vi "Cavities_Pulse_FPGA_v00.vi"() -> ()   [LabVIEW 2010]
doc: "Four cavities are controlled here:\n1) OPO A\n2) OPO B\n3) mode Cleaner\n4) Doubler\nThe output can either be Scanned, Locked, or Held."
uses:
  Strict Type Defs/Scope.ctl
  Strict Type Defs/Pulse Control.ctl
  Strict Type Defs/Cavity Errors.ctl
  Strict Type Defs/Cavity Monitors.ctl
  Strict Type Defs/Zero Crossing.ctl
  Strict Type Defs/Control.ctl
  Strict Type Defs/PII individual.ctl
  Strict Type Defs/Safety First.ctl
  Strict Type Defs/Error Scale.ctl
  Strict Type Defs/Lock Thresh.ctl
  <vilib>/eio/EIONode/EIONode.xnode
  <vilib>/rvi/eio/nirviEIOImplementation/nirviEIOImplementation.xnode
  <vilib>/rvi/eio/common/nirviEmuClasses.ctl
  <vilib>/rvi/DataTransferAndStorage/Container/XNode/niFpgaContainer.xnode
  <vilib>/rvi/DataTransferAndStorage/Container/Common/niFpgaContainerMethod.ctl
  <vilib>/rvi/DataTransferAndStorage/Container/Common/niFpgaTransferTypeControl.ctl
  <vilib>/rvi/eio/common/nirviEmuTemplateMethod_noerrors.vi
  <vilib>/rvi/interface/RandomDataEmulation/nirviRandomDataFPGAFIFO.vi
  <vilib>/rvi/interface/RandomDataEmulation/niFpgaRandomDataHandleErrors.vi
panel:
  in  "quit Control Loop":bool
  in  "Control":T1={"PII In 1"={"Lock"=FALSE, "Hold"=FALSE, "P Gain"=0, "P BS"=-5, "I Gain"=0, "I BS"=-10, "I2 G"=0, "I2 BS"=-26, "Scan Amp"=0, "Scan Off"=0, "Scan FS"=0, "SFS BS"=0, "I Max value"=10000, "I2 Max value"=10000, "Scope.Offset"=0, "Trigger Direction"=enum."either", "Scan-PII thresh"=0}, "PII In 2"={"Lock"=FALSE, "Hold"=FALSE, "P Gain"=0, "P BS"=-10, "I Gain"=0, "I BS"=-10, "I2 G"=0, "I2 BS"=-26, "Scan Amp"=0, "Scan Off"=0, "Scan FS"=0, "SFS BS"=0, "I Max value"=10000, "I2 Max value"=10000, "Scope.Offset"=0, "Trigger Direction"=enum."either", "Scan-PII thresh"=0}, "PII In 3"={"Lock"=FALSE, "Hold"=FALSE, "P Gain"=0, "P BS"=-10, "I Gain"=0, "I BS"=-10, "I2 G"=0, "I2 BS"=-26, "Scan Amp"=0, "Scan Off"=0, "Scan FS"=0, "SFS BS"=0, "I Max value"=10000, "I2 Max value"=10000, "Scope.Offset"=0, "Trigger Direction"=enum."either", "Scan-PII thresh"=0}, "PII In 4"={"Lock"=FALSE, "Hold"=FALSE, "P Gain"=0, "P BS"=-10, "I Gain"=0, "I BS"=-10, "I2 G"=0, "I2 BS"=-26, "Scan Amp"=0, "Scan Off"=0, "Scan FS"=0, "SFS BS"=0, "I Max value"=10000, "I2 Max value"=10000, "Scope.Offset"=0, "Trigger Direction"=enum."either", "Scan-PII thresh"=0}, "Safety First"={"lim reset"=FALSE, "no limit"=FALSE, "pos slew rate * dt"=10, "neg slew rate * dt"=-10, "Hold All"=FALSE, "Count(Ticks)"=0}, "Error scale"={"Pre-Offset"={"Pre-Offset 1"=2, "Pre-Offset 2"=0, "Pre-Offset 3"=0, "Pre-Offset 4"=0, "Pre-Offset 5"=2, "Pre-Offset 6"=0, "Pre-Offset 7"=0, "Pre-Offset 8"=0}, "Post-Offset "={"Offset 1"=0, "Offset 2"=300, "Offset 3"=0, "Offset 4"=0, "Offset 5"=0, "Offset 6"=0, "Offset 7"=0, "Offset 8"=0}, "Gains"={"Gain 1"=0, "Gain 2"=300, "Gain 3"=0, "Gain 4"=0, "Gain 5"=0, "Gain 6"=0, "Gain 7"=0, "Gain 8"=0}, "Polarity DC"={"False 1"=FALSE, "False 2"=FALSE, "False 3"=FALSE, "False 4"=FALSE, "DC x -1"=FALSE, "DC x -1 2"=FALSE, "DC x -1 3"=FALSE, "DC x -1 4"=FALSE}}, "Lock Thresh"={"OPO A"=2, "OPO B"=0, "MCC"=40, "Doubler"=0}, "Re-Scan Thresh"={"OPO A"=0, "OPO B"=0, "MCC"=0, "Doubler"=0}}
  in  "\"I too high?\"":T6
  in  "\"Outputs\"":T7
  out "Outputs":T8={"OPO A out"=-270, "OPO B out"=-1710, "MCC out"=880, "Doubler out"=570}
  in  "\"Trigger\"":T9
  out "Trigger":T9
  out "Cavity Monitors":T10
  out "Cavity Errors":T11={"OPO A"=0, "OPO B"=1800, "MCC"=0, "Doubler"=0}
  out "Control Loop count":i32=11285327
  out "Lock Threshold":T12
  in  "Cavities Delay(uSec)":u32 caption="Count(uSec)"
  in  "Lock Monitor":T7
  out "Unlocked?(T=yes)":T6
  in  "RMS Stop":bool
  out "RMS Count":i32
  in  "Measurement OFF (uSec)":u32 caption="Measurement OFF(uSec)"
  in  "offset time":u32
  out "Measurement Tick Count(uSec)":u32
  out "PXI Trig 2":bool
  in  "Measurement OFF":bool
  out "Pulse large loop count":i32
  in  "Pulse Loop On":bool
  in  "stop pulse loop":bool
  out "Pulse Loop count":i32
  out "Tick Count(uSec)":u32
  out "BS Hold Pulse":bool
  out "Probe OFF Pulse":bool
  out "HD Pulse":bool
  out "Measurment Pulse":bool
  in  "Pulse Control":T13
  in  "Scope":T14={"Trigger Direction"=enum."plus-minus", "Delay"=0, "Aquisition Rate (Ticks)"=40, "Offset"=0, "Channel"=0, "Channel Selector"={"Channel 1"=0, "Channel 2"=4, "Channel 3"=8, "Channel 4"=8}} {"Channel Selector"."Channel 4" items=["Error Signal 1", "Error Signal 2", "Scan Trigger 1", "Scan Trigger 2", "DC Signal 1", "DC Signal 2", "PI Out 1", "PI Out 2"]; "Channel Selector"."Channel 3" items=["Error Signal 1", "Error Signal 2", "Scan Trigger 1", "Scan Trigger 2", "DC Signal 1", "DC Signal 2", "PI Out 1", "PI Out 2"]; "Channel Selector"."Channel 2" items=["Error Signal 1", "Error Signal 2", "Scan Trigger 1", "Scan Trigger 2", "DC Signal 1", "DC Signal 2", "PI Out 1", "PI Out 2"]; "Channel Selector"."Channel 1" items=["Error Signal 1", "Error Signal 2", "Scan Trigger 1", "Scan Trigger 2", "DC Signal 1", "DC Signal 2", "PI Out 1", "PI Out 2"]}
  out "Scope Full?":bool
  out "Scope loop count":i32=119818
  # "All time values are in micro-seconds"
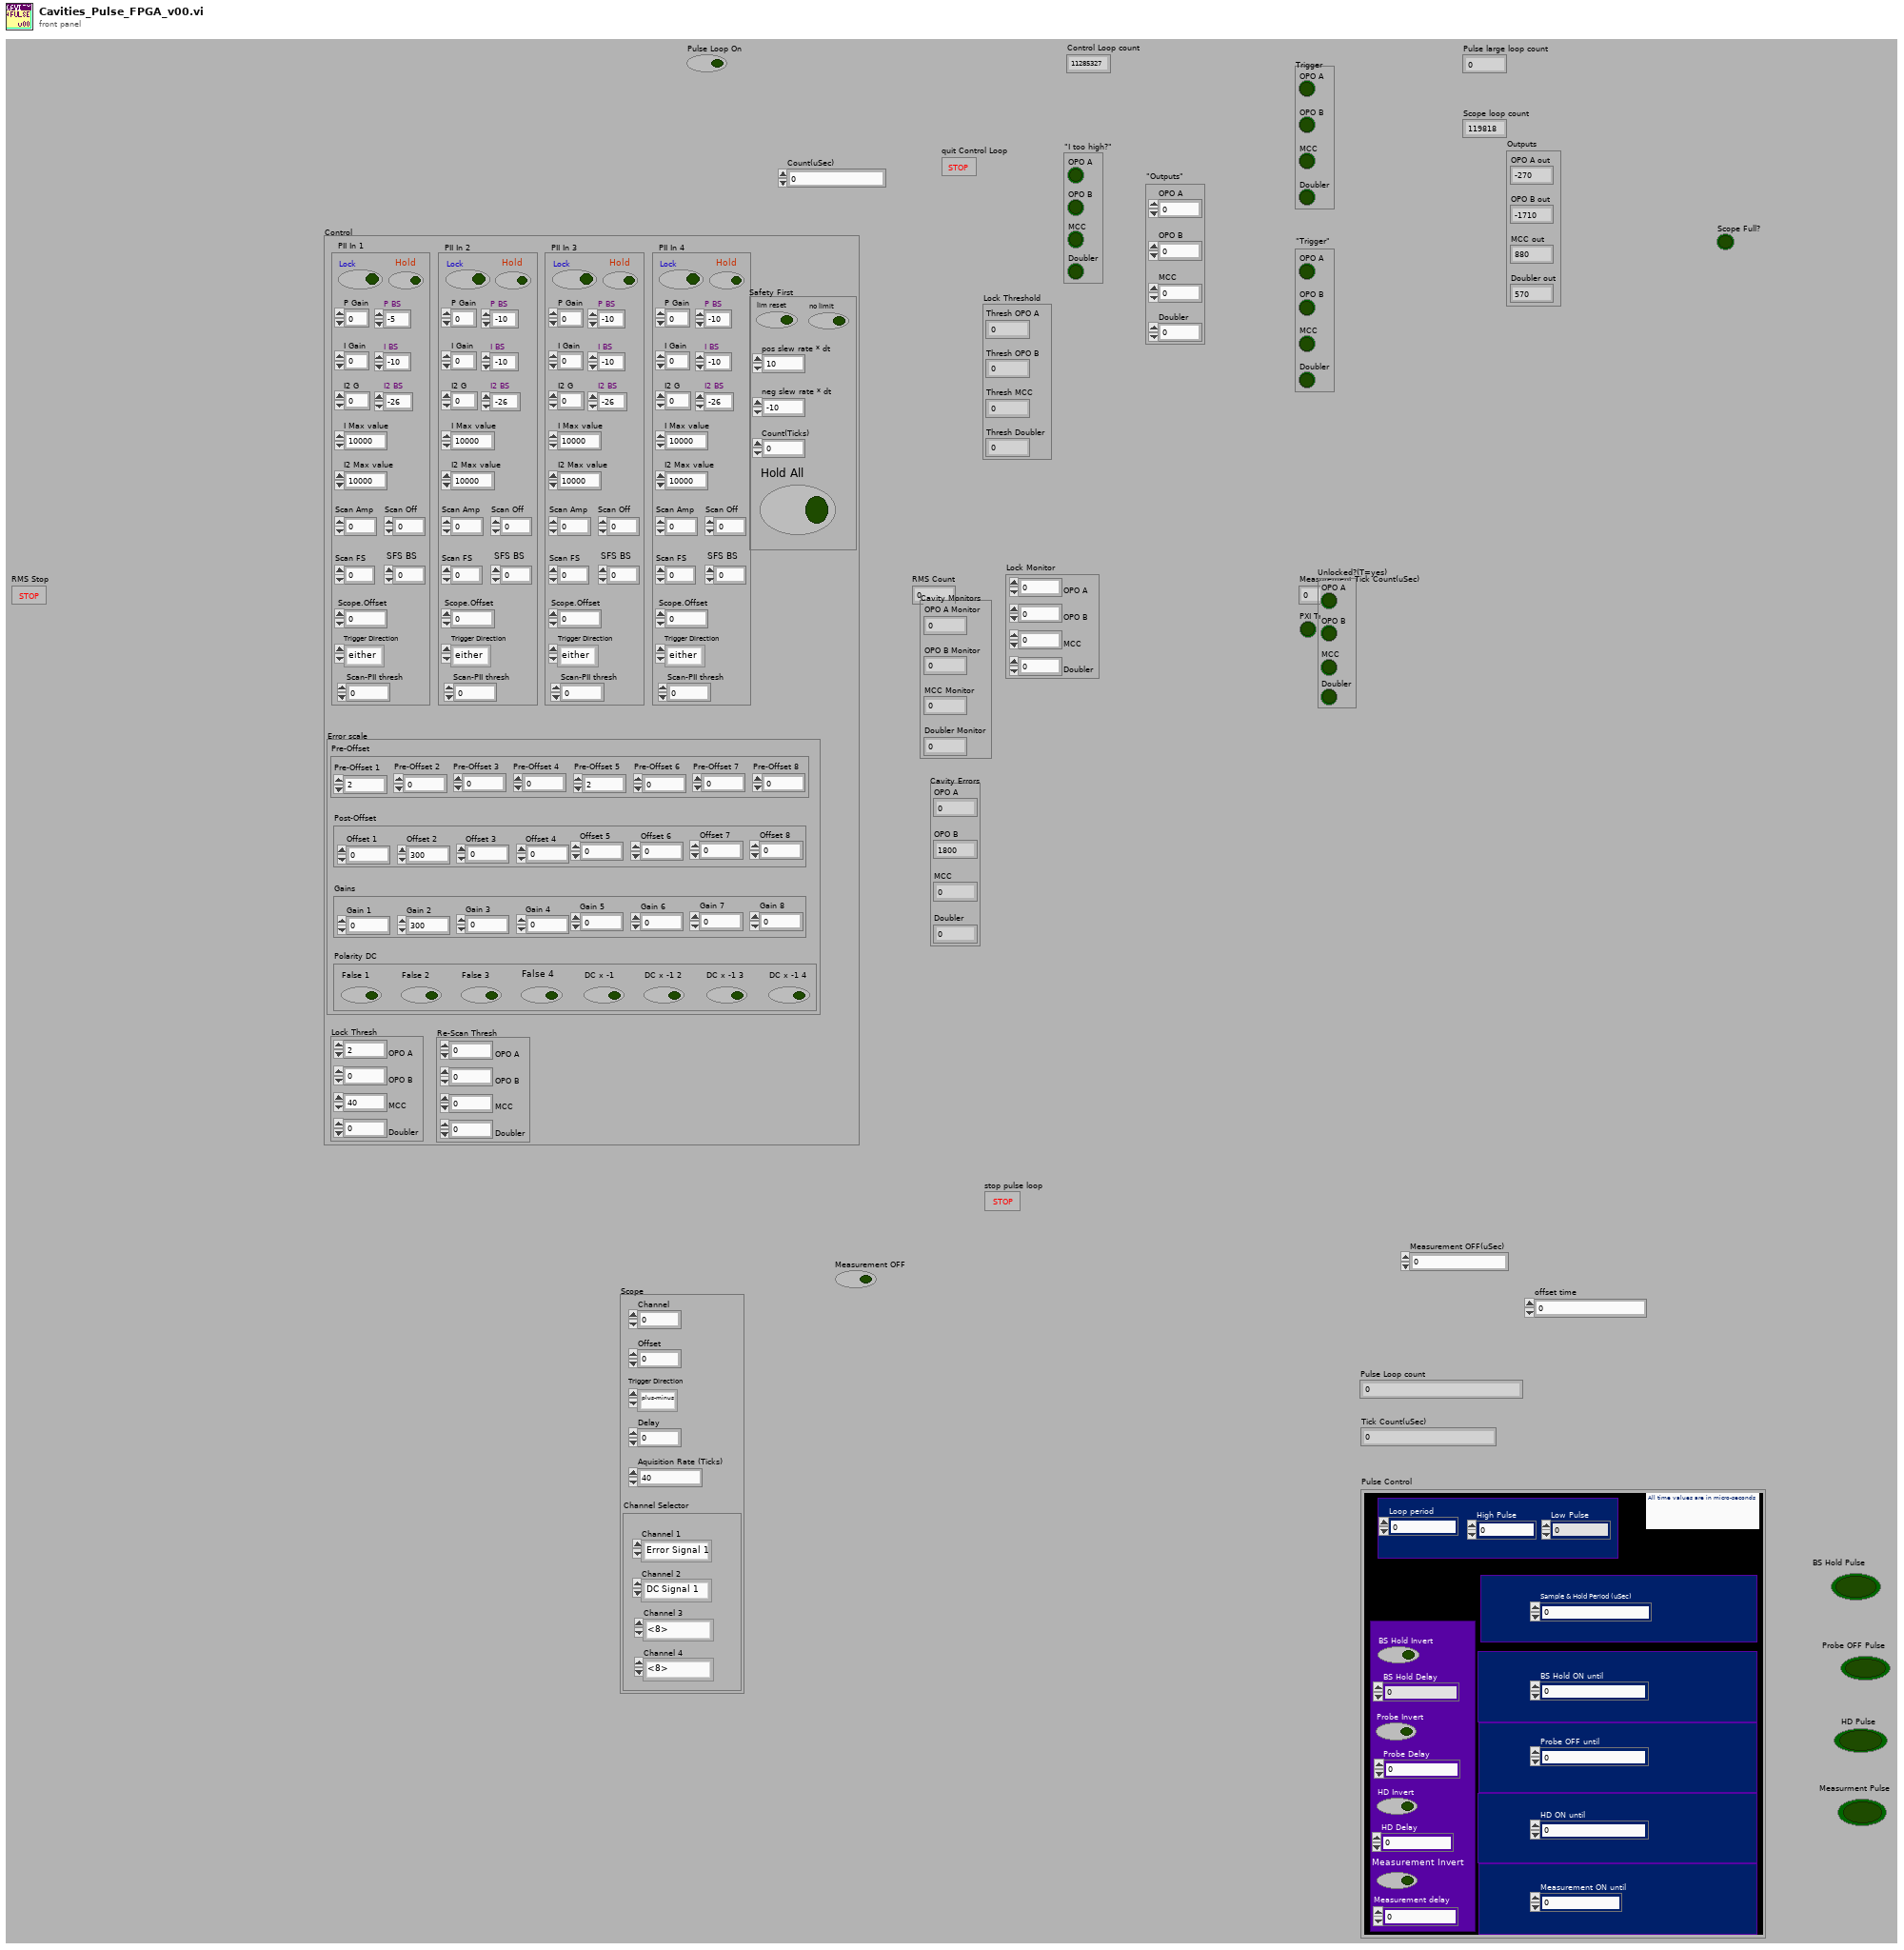
[diagram p1: front panel]
types:
  T1 = typedef "Control.ctl" = cluster{"PII In 1":T2, "PII In 2":T2, "PII In 3":T2, "PII In 4":T2, "Safety First":T3, "Error scale":T4, "Lock Thresh":T5, "Re-Scan Thresh":T5}
  T2 = typedef "PII individual.ctl" = cluster{"Lock":bool, "Hold":bool, "P Gain":i32, "P BS":i16, "I Gain":i32, "I BS":i16, "I2 G":i32, "I2 BS":i16, "Scan Amp":i16, "Scan Off":i16, "Scan FS":u16, "SFS BS":i16, "I Max value":i32, "I2 Max value":i32, "Scope.Offset":i16, "Trigger Direction":enum8{"either", "minus-plus", "plus-minus"}, "Scan-PII thresh":i16}
  T3 = typedef "Safety First.ctl" = cluster{"lim reset":bool, "no limit":bool, "pos slew rate * dt":i16, "neg slew rate * dt":i16, "Hold All":bool, "Count(Ticks)":u32}
  T4 = typedef "Error Scale.ctl" = cluster{"Pre-Offset":cluster{"Pre-Offset 1":i16, "Pre-Offset 2":i16, "Pre-Offset 3":i16, "Pre-Offset 4":i16, "Pre-Offset 5":i16, "Pre-Offset 6":i16, "Pre-Offset 7":i16, "Pre-Offset 8":i16}, "Post-Offset ":cluster{"Offset 1":i16, "Offset 2":i16, "Offset 3":i16, "Offset 4":i16, "Offset 5":i16, "Offset 6":i16, "Offset 7":i16, "Offset 8":i16}, "Gains":cluster{"Gain 1":i16, "Gain 2":i16, "Gain 3":i16, "Gain 4":i16, "Gain 5":i16, "Gain 6":i16, "Gain 7":i16, "Gain 8":i16}, "Polarity DC":cluster{"False 1":bool, "False 2":bool, "False 3":bool, "False 4":bool, "DC x -1":bool, "DC x -1 2":bool, "DC x -1 3":bool, "DC x -1 4":bool}}
  T5 = typedef "Lock Thresh.ctl" = cluster{"OPO A":i16, "OPO B":i16, "MCC":i16, "Doubler":i16}
  T6 = cluster{"OPO A":bool, "OPO B":bool, "MCC":bool, "Doubler":bool}
  T7 = cluster{"OPO A":i16, "OPO B":i16, "MCC":i16, "Doubler":i16}
  T8 = cluster{"OPO A out":i16, "OPO B out":i16, "MCC out":i16, "Doubler out":i16}
  T9 = typedef "Zero Crossing.ctl" = cluster{"OPO A":bool, "OPO B":bool, "MCC":bool, "Doubler":bool}
  T10 = typedef "Cavity Monitors.ctl" = cluster{"OPO A Monitor":i16, "OPO B Monitor":i16, "MCC Monitor":i16, "Doubler Monitor":i16}
  T11 = typedef "Cavity Errors.ctl" = cluster{"OPO A":i16, "OPO B":i16, "MCC":i16, "Doubler":i16}
  T12 = cluster{"Thresh OPO A ":i16, "Thresh OPO B":i16, "Thresh MCC":i16, "Thresh Doubler":i16}
  T13 = typedef "Pulse Control.ctl" = cluster{"BS Hold Invert":bool, "Probe Invert":bool, "HD Invert":bool, "Measurement Invert":bool, "BS Hold Delay":u32, "Probe Delay":u32, "HD Delay":u32, "Measurement delay":u32, "High Pulse":i16, "Low Pulse":i16, "Sample & Hold Period (uSec)":u32, "BS Hold ON until":u32, "Probe OFF until":u32, "HD ON until":u32, "Measurement ON until":u32, "Loop period (us)":u16}
  T14 = typedef "Scope.ctl" = cluster{"Trigger Direction":enum8{"either", "minus-plus", "plus-minus"}, "Delay":u32, "Aquisition Rate (Ticks)":u32, "Offset":i16, "Channel":i32, "Channel Selector":cluster{"Channel 1":i32, "Channel 2":i32, "Channel 3":i32, "Channel 4":i32}}
  T15 = typedef "nirviEmuClasses.ctl" = enum16{"IO Read", "IO Write", "Method", "Property Read", "Property Write"}
  T16 = typedef "Signals.ctl" = cluster{"Cavity Errors":T11, "Cavity Monitors":T10, "Lock Thresh":T5, "Re-Scan Thresh":T5, "PII In 1":T2, "PII In 2":T2, "PII In 3":T2, "PII In 4":T2, "Safety First":T3}
  T17 = typedef "Control Cavity Cluster.ctl" = cluster{"Control A":T2, "Control B":T2, "Control MCC":T2, "Control Doubler":T2, "Lock Point?":T18, "Re-scan?":T19, "Cavity Errors":T11, "Max":T20, "Min":T21, "Lock Threshold":cluster{"Thresh OPO A ":i16, "Thresh OPO B":i16, "Thresh MCC":i16, "Thresh Doubler":i16}, "Re-Scan Threshold":cluster{"Thresh OPO A ":i16, "Thresh OPO B":i16, "Thresh MCC":i16, "Thresh Doubler":i16}, "State (-1)":cluster{"OPO A":enum16{"Safe", "Hold", "Scan", "Lock"}, "OPO B":enum16{"Safe", "Hold", "Scan", "Lock"}, "MCC":enum16{"Safe", "Hold", "Scan", "Lock"}, "Doubler":enum16{"Safe", "Hold", "Scan", "Lock"}}, "Lock pressed? (-1)":cluster{"OPO A":bool, "OPO B":bool, "MCC":bool, "Doubler":bool}, "Safety First":T3}
  T18 = typedef "Lock Point.ctl" = cluster{"OPO A":bool, "OPO B":bool, "MCC":bool, "Doubler":bool}
  T19 = typedef "Re-Scan.ctl" = cluster{"OPO A":bool, "OPO B":bool, "MCC":bool, "Doubler":bool}
  T20 = typedef "Max.ctl" = cluster{"Max OPO A":i16, "Max OPO B":i16, "Max MCC":i16, "Max Doubler":i16}
  T21 = typedef "Min.ctl" = cluster{"Min OPO A":i16, "Min OPO B":i16, "Min MCC":i16, "Min Doubler":i16}
  T22 = typedef "PII Scan State.ctl" = cluster{"Control A":T2, "Control B":T2, "Control MCC":T2, "Control Doubler":T2, "Cavity Errors":T11, "State":cluster{"OPO A":enum16{"Safe", "Hold", "Scan", "Lock"}, "OPO B":enum16{"Safe", "Hold", "Scan", "Lock"}, "MCC":enum16{"Safe", "Hold", "Scan", "Lock"}, "Doubler":enum16{"Safe", "Hold", "Scan", "Lock"}}}
  T23 = typedef "MaxMin.ctl" = cluster{"State":cluster{"OPO A":enum16{"Safe", "Hold", "Scan", "Lock"}, "OPO B":enum16{"Safe", "Hold", "Scan", "Lock"}, "MCC":enum16{"Safe", "Hold", "Scan", "Lock"}, "Doubler":enum16{"Safe", "Hold", "Scan", "Lock"}}, "Reset MaxMin?":cluster{"OPO A":bool, "OPO B":bool, "MCC":bool, "Doubler":bool}, "Max":T20, "Min":T21, "Lock pressed?":cluster{"OPO A":bool, "OPO B":bool, "MCC":bool, "Doubler":bool}, "Safety First":T3}
  T24 = typedef "niFpgaContainerMethod.ctl" = enum16{"<none>", "write", "read", "clear", "getNumberOfElementsToWrite", "getNumberOfElementsToRead", "enable", "disable", "flushAndDisable", "getStreamState", "readA", "readB", "dramWrite", "dramWriteWithByteEnables", "dramRequestData", "dramRetrieveData"}
  T25 = typedef "niFpgaTransferTypeControl.ctl" = enum16{"Target-Scoped", "Host to Target - DMA", "Target to Host - DMA", "Peer to Peer Reader", "Peer to Peer Writer", "Bidirectional"}
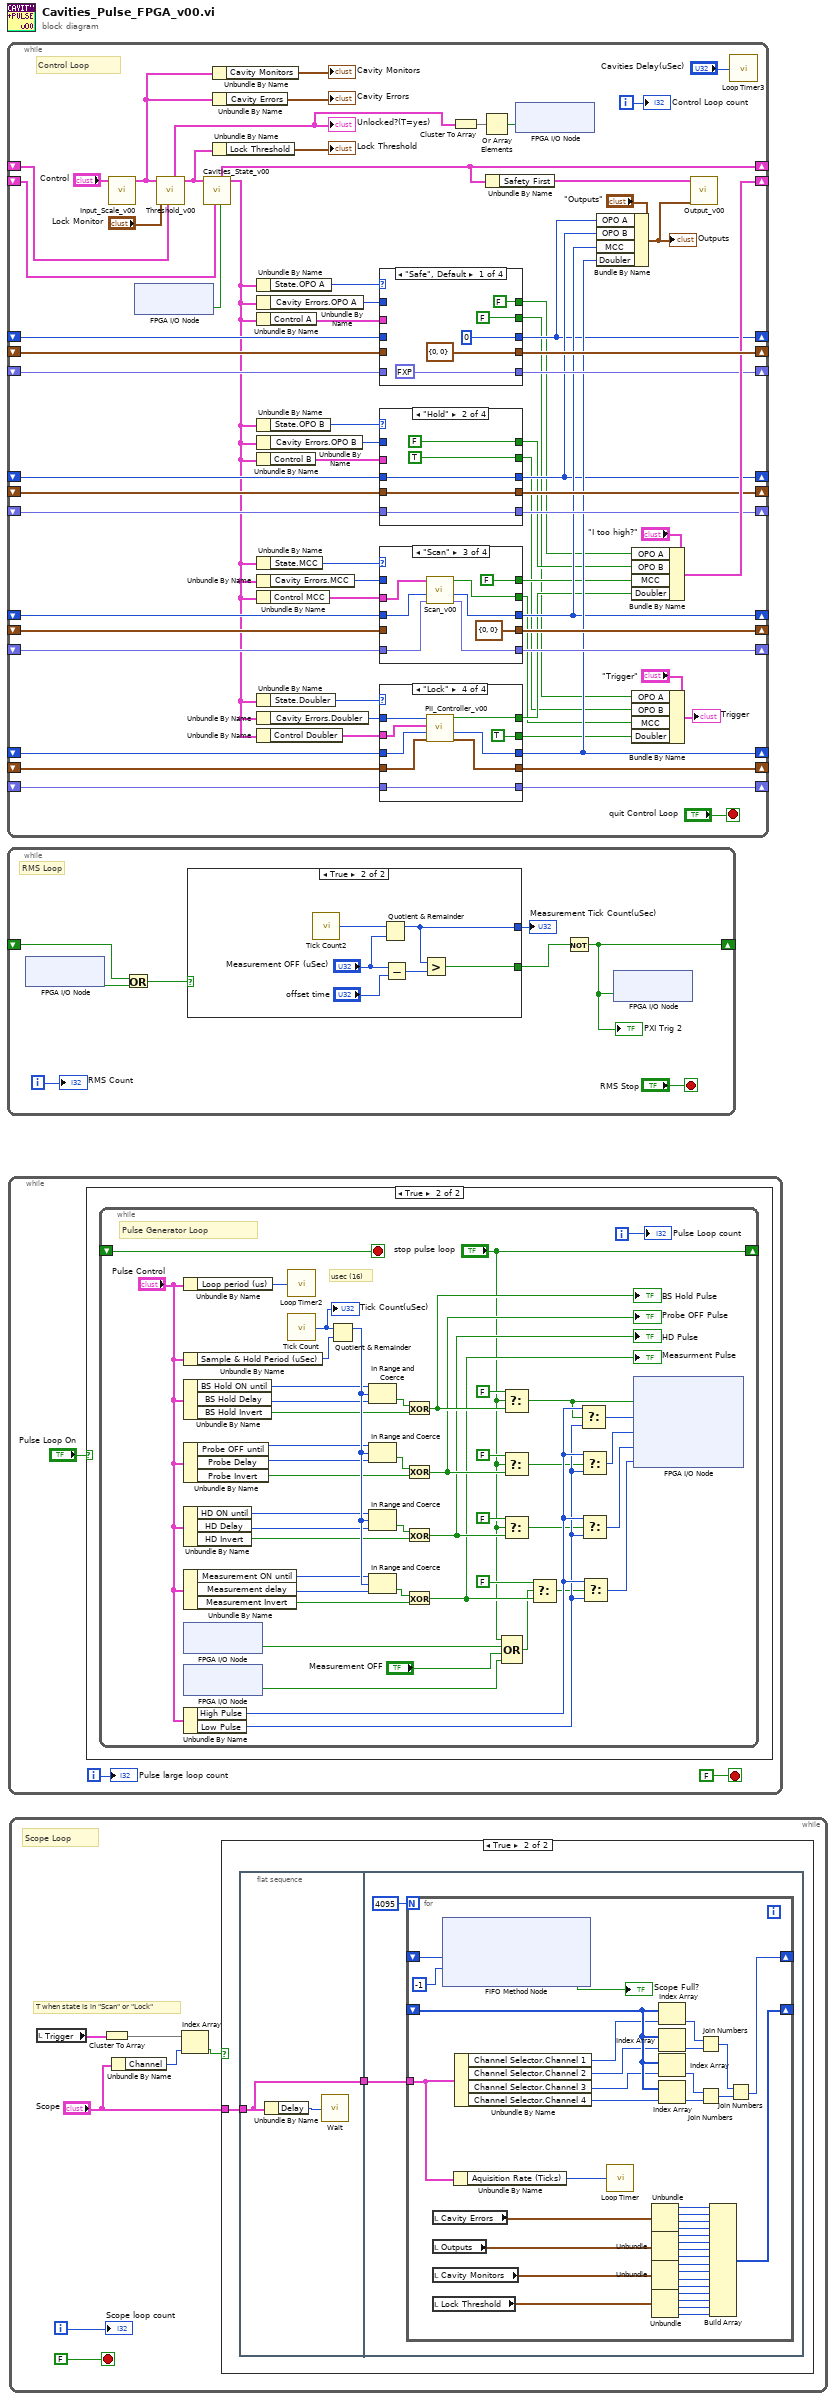
[diagram p0: block diagram]
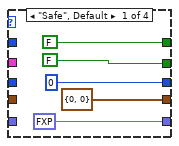
[diagram p2: hidden frame]
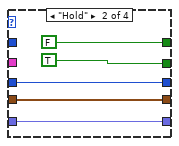
[diagram p3: hidden frame]
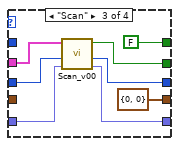
[diagram p4: hidden frame]
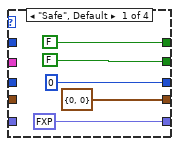
[diagram p5: hidden frame]
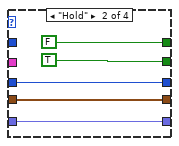
[diagram p6: hidden frame]
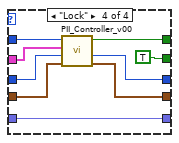
[diagram p7: hidden frame]
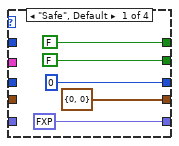
[diagram p8: hidden frame]
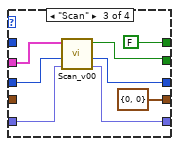
[diagram p9: hidden frame]
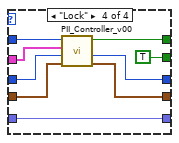
[diagram p10: hidden frame]
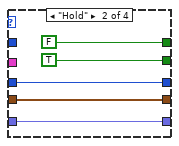
[diagram p11: hidden frame]
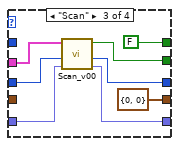
[diagram p12: hidden frame]
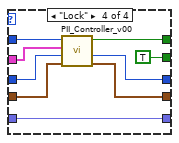
[diagram p13: hidden frame]
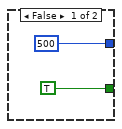
[diagram p14: hidden frame]
diagram:
  n1 = while {
    shift-right: [w68] -> _
    shift-left: _ -> [w66]
    shift-right: [w65] -> _
    shift-left: _ -> [w5]
    shift-right: [w34] -> _
    shift-left: _ -> [w67]
    shift-right: [w62] -> _
    shift-left: _ -> [w61]
    shift-right: [w40] -> _
    shift-left: _ -> [w6]
    shift-right: [w51] -> _
    shift-left: _ -> [w53]
    shift-right: [w35] -> _
    shift-left: _ -> [w52]
    shift-right: [w54] -> _
    shift-left: _ -> [w55]
    shift-right: [w50] -> _
    shift-left: _ -> [w48]
    shift-right: [w36] -> _
    shift-left: _ -> [w49]
    shift-right: [w47] -> _
    shift-left: _ -> [w46]
    shift-right: [w41] -> _
    shift-left: _ -> [w43]
    shift-right: [w37] -> _
    shift-left: _ -> [w42]
    shift-right: [w44] -> _
    shift-left: _ -> [w45]
    i -> [w58]
    stop <- "quit Control Loop" stop-if-true
    # "Control Loop"
    n2 = call "Input_Scale_v00.vi"("Control"="Control") -> ("Signals"=w22:T16)  [unwired: 10 in]
    n3 = xnode "FPGA I/O Node"() -> ("PXI_Trig0"=w4:bool)  [unwired: 1 in, 1 out]
    n4 = call "Threshold_v00.vi"("MaxMin"=w6, "Lock Monitor"="Lock Monitor", "Signals"=w22) -> ("Control Cavity Cluster"=w26:T17, "Unlocked?(T=yes)"=w1:T6)  [unwired: 7 in]
    "Unlocked?(T=yes)" <- w1
    n5 = call "Cavities_State_v00.vi"("BS Hold Pulse"=w4, "\"I too high?\""=w5, "Control Cavity Cluster"=w26) -> ("PII Scan State Errors"=w7:T22, "MaxMin"=w40:T23)  [unwired: 7 in]
    n6 = Unbundle By Name(w22) -> ("Cavity Monitors"=→"Cavity Monitors":T10)
    n7 = Unbundle By Name(w22) -> ("Cavity Errors"=→"Cavity Errors":T11)
    n8 = Unbundle By Name(w26) -> ("Lock Threshold"=→"Lock Threshold":T12)
    n9 = Unbundle By Name(w7) -> ("State.OPO A"=w56:enum16{"Safe", "Hold", "Scan", "Lock"})
    n10 = Unbundle By Name(w7) -> ("Cavity Errors.OPO A"=w17:i16)
    n11 = Unbundle By Name(w7) -> ("Control A"=w18:T2)
    n12 = Unbundle By Name(w7) -> ("State.OPO B"=w15:enum16{"Safe", "Hold", "Scan", "Lock"})
    n13 = Unbundle By Name(w7) -> ("Cavity Errors.OPO B"=w16:i16)
    n14 = Unbundle By Name(w7) -> ("Control B"=w14:T2)
    n15 = Unbundle By Name(w7) -> ("State.MCC"=w13:enum16{"Safe", "Hold", "Scan", "Lock"})
    n16 = Unbundle By Name(w7) -> ("Cavity Errors.MCC"=w12:i16)
    n17 = Unbundle By Name(w7) -> ("Control MCC"=w11:T2)
    n18 = Unbundle By Name(w7) -> ("State.Doubler"=w10:enum16{"Safe", "Hold", "Scan", "Lock"})
    n19 = Unbundle By Name(w7) -> ("Cavity Errors.Doubler"=w9:i16)
    n20 = Unbundle By Name(w7) -> ("Control Doubler"=w8:T2)
    n21 = case shown="\"Safe\", Default" w56 {
      tunnel: w17 -> [_ _ _ w207]
      tunnel: [cluster{"I Cavity":i32, "I2 Cavity":i32} {"I Cavity"=0, "I2 Cavity"=0} ("Integrator") w188 cluster{"I Cavity":i32, "I2 Cavity":i32} {"I Cavity"=0, "I2 Cavity"=0} ("Integrator") w203] -> w68
      tunnel: [FALSE ("I too high? (F=No)") FALSE ("I too high? (F=No)") FALSE ("I too high? (F=No)") w206] -> w33
      tunnel: w18 -> [_ _ w197 w204]
      tunnel: [i16 0 ("PII out") w189 w196 w200] -> w34
      tunnel: w67 -> [_ w189 w193 w201]
      tunnel: w66 -> [_ w188 _ w205]
      tunnel: [fxp<+,33,17> 0.0 ("Scan") w187 w195 w199] -> w62
      tunnel: w61 -> [_ w187 w194 w199]
      tunnel: [FALSE ("Zero Crossing") TRUE ("Zero Crossing") w192 TRUE ("Zero Crossing")] -> w29
      frame "Safe", Default {
      }
      frame "Hold" {
      }
      frame "Scan" {
        n22 = call "Scan_v00.vi"("Scan (-1)"=w194, "Scan out (-1)"=w193, "Control Cavity"=w197) -> ("Scan"=w195:fxp<+,33,17>, "Scan out"=w196:i16, "Zero Crossing"=w192:bool)  [unwired: 6 in]
      }
      frame "Lock" {
        n23 = call "PII_Controller_v00.vi"("Integrator (-1)"=w205, "PII out (-1)"=w201, "Control Cavity"=w204, "OPO A Error"=w207) -> ("Integrator"=w203:cluster{"I Cavity":i32, "I2 Cavity":i32}, "PII out"=w200:i16, "I too high?"=w206:bool)  [unwired: 5 in]
      }
    }
    n24 = case shown="\"Hold\"" w15 {
      tunnel: w16 -> [_ _ _ w180]
      tunnel: [cluster{"I Cavity":i32, "I2 Cavity":i32} {"I Cavity"=0, "I2 Cavity"=0} ("Integrator") w161 cluster{"I Cavity":i32, "I2 Cavity":i32} {"I Cavity"=0, "I2 Cavity"=0} ("Integrator") w176] -> w51
      tunnel: [FALSE ("I too high? (F=No)") FALSE ("I too high? (F=No)") FALSE ("I too high? (F=No)") w179] -> w32
      tunnel: w14 -> [_ _ w170 w177]
      tunnel: [i16 0 ("PII out") w162 w169 w174] -> w35
      tunnel: w52 -> [_ w162 w166 w175]
      tunnel: w53 -> [_ w161 _ w178]
      tunnel: [fxp<+,33,17> 0.0 ("Scan") w160 w168 w173] -> w54
      tunnel: w55 -> [_ w160 w167 w173]
      tunnel: [FALSE ("Zero Crossing") TRUE ("Zero Crossing") w164 TRUE ("Zero Crossing")] -> w21
      frame "Safe", Default {
      }
      frame "Hold" {
      }
      frame "Scan" {
        n25 = call "Scan_v00.vi"("Scan (-1)"=w167, "Scan out (-1)"=w166, "Control Cavity"=w170) -> ("Scan"=w168:fxp<+,33,17>, "Scan out"=w169:i16, "Zero Crossing"=w164:bool)  [unwired: 6 in]
      }
      frame "Lock" {
        n26 = call "PII_Controller_v00.vi"("Integrator (-1)"=w178, "PII out (-1)"=w175, "Control Cavity"=w177, "OPO A Error"=w180) -> ("Integrator"=w176:cluster{"I Cavity":i32, "I2 Cavity":i32}, "PII out"=w174:i16, "I too high?"=w179:bool)  [unwired: 5 in]
      }
    }
    n27 = case shown="\"Scan\"" w13 {
      tunnel: w12 -> [_ _ _ w153]
      tunnel: [cluster{"I Cavity":i32, "I2 Cavity":i32} {"I Cavity"=0, "I2 Cavity"=0} ("Integrator") w134 cluster{"I Cavity":i32, "I2 Cavity":i32} {"I Cavity"=0, "I2 Cavity"=0} ("Integrator") w149] -> w50
      tunnel: [FALSE ("I too high? (F=No)") FALSE ("I too high? (F=No)") FALSE ("I too high? (F=No)") w152] -> w31
      tunnel: w11 -> [_ _ w143 w150]
      tunnel: [i16 0 ("PII out") w135 w142 w146] -> w36
      tunnel: w49 -> [_ w135 w139 w147]
      tunnel: w48 -> [_ w134 _ w151]
      tunnel: [fxp<+,33,17> 0.0 ("Scan") w133 w141 w145] -> w47
      tunnel: w46 -> [_ w133 w140 w145]
      tunnel: [FALSE ("Zero Crossing") TRUE ("Zero Crossing") w138 TRUE ("Zero Crossing")] -> w28
      frame "Safe", Default {
      }
      frame "Hold" {
      }
      frame "Scan" {
        n28 = call "Scan_v00.vi"("Scan (-1)"=w140, "Scan out (-1)"=w139, "Control Cavity"=w143) -> ("Scan"=w141:fxp<+,33,17>, "Scan out"=w142:i16, "Zero Crossing"=w138:bool)  [unwired: 6 in]
      }
      frame "Lock" {
        n29 = call "PII_Controller_v00.vi"("Integrator (-1)"=w151, "PII out (-1)"=w147, "Control Cavity"=w150, "OPO A Error"=w153) -> ("Integrator"=w149:cluster{"I Cavity":i32, "I2 Cavity":i32}, "PII out"=w146:i16, "I too high?"=w152:bool)  [unwired: 5 in]
      }
    }
    n30 = case shown="\"Lock\"" w10 {
      tunnel: w9 -> [_ _ _ w126]
      tunnel: [cluster{"I Cavity":i32, "I2 Cavity":i32} {"I Cavity"=0, "I2 Cavity"=0} ("Integrator") w107 cluster{"I Cavity":i32, "I2 Cavity":i32} {"I Cavity"=0, "I2 Cavity"=0} ("Integrator") w122] -> w41
      tunnel: [FALSE ("I too high? (F=No)") FALSE ("I too high? (F=No)") FALSE ("I too high? (F=No)") w125] -> w30
      tunnel: w8 -> [_ _ w116 w123]
      tunnel: [i16 0 ("PII out") w108 w115 w119] -> w37
      tunnel: w42 -> [_ w108 w112 w120]
      tunnel: w43 -> [_ w107 _ w124]
      tunnel: [fxp<+,33,17> 0.0 ("Scan") w106 w114 w118] -> w44
      tunnel: w45 -> [_ w106 w113 w118]
      tunnel: [FALSE ("Zero Crossing") TRUE ("Zero Crossing") w111 TRUE ("Zero Crossing")] -> w27
      frame "Safe", Default {
      }
      frame "Hold" {
      }
      frame "Scan" {
        n31 = call "Scan_v00.vi"("Scan (-1)"=w113, "Scan out (-1)"=w112, "Control Cavity"=w116) -> ("Scan"=w114:fxp<+,33,17>, "Scan out"=w115:i16, "Zero Crossing"=w111:bool)  [unwired: 6 in]
      }
      frame "Lock" {
        n32 = call "PII_Controller_v00.vi"("Integrator (-1)"=w124, "PII out (-1)"=w120, "Control Cavity"=w123, "OPO A Error"=w126) -> ("Integrator"=w122:cluster{"I Cavity":i32, "I2 Cavity":i32}, "PII out"=w119:i16, "I too high?"=w125:bool)  [unwired: 5 in]
      }
    }
    n33 = Cluster To Array(cluster=w1) -> (array=w3:bool[])
    n34 = Or Array Elements(Boolean array=w3) -> (logical OR=w2:bool)
    n35 = Unbundle By Name(w40) -> ("Safety First"=w39:T3)
    n36 = xnode "FPGA I/O Node"("PXI_Trig3"=w2) -> ()  [unwired: 1 in, 1 out]
    n37 = Bundle By Name(cluster="\"Outputs\"", "OPO A"=w34, "OPO B"=w35, "MCC"=w36, "Doubler"=w37) -> (w38:T7)
    "Outputs" <- w38
    n38 = Bundle By Name(cluster="\"I too high?\"", "OPO A"=w33, "OPO B"=w32, "MCC"=w31, "Doubler"=w30) -> (w65:T6)
    n39 = Bundle By Name(cluster="\"Trigger\"", "OPO A"=w29, "OPO B"=w21, "MCC"=w28, "Doubler"=w27) -> (→"Trigger":T9)
    n40 = call "Output_v00.vi"("Outputs"=w38, "Safety First"=w39) -> ()  [unwired: 10 in]
    n41 = call "Loop Timer3"("Count(uSec)"="Cavities Delay(uSec)") -> ()  [unwired: 1 out]
    "Control Loop count" <- w58
  }
  n42 = while {
    shift-right: [w209] -> _
    shift-left: _ -> [w211]
    i -> [w214]
    stop <- "RMS Stop" stop-if-true
    # "RMS Loop"
    n43 = xnode "FPGA I/O Node"() -> ("PXI_Trig3"=w208:bool)  [unwired: 1 in, 1 out]
    n44 = Or(x=w211, y=w208) -> (x .or. y?=w213:bool)
    n45 = case shown="True" w213 {
      tunnel: [TRUE ("t") w237] -> w212
      tunnel: [u32 500 ("Tick Count(uSec)") w241] -> w210
      frame False {
      }
      frame True {
        n46 = call "Tick Count2"() -> ("Tick Count(uSec)"=w242:u32)
        n47 = Quotient & Remainder(x=w242, y="Measurement OFF (uSec)") -> (x-y*floor(x/y)=w241:u32)  [unwired: 1 out]
        n48 = Subtract(x="Measurement OFF (uSec)", y="offset time") -> (x-y=w238:u32)
        n49 = Greater?(x=w241, y=w238) -> (0:w237:bool)
      }
    }
    "Measurement Tick Count(uSec)" <- w210
    n50 = Not(x=w212) -> (.not. x?=w209:bool)
    "PXI Trig 2" <- w209
    n51 = xnode "FPGA I/O Node"("PXI_Trig2"=w209) -> ()  [unwired: 1 in, 1 out]
    "RMS Count" <- w214
  }
  n52 = while {
    i -> [w255]
    stop <- FALSE stop-if-true
    n53 = case shown="True" "Pulse Loop On" {
      frame False {
      }
      frame True {
        n54 = while {
          shift-right: ["stop pulse loop"] -> _
          shift-left: _ -> [w263]
          i -> [w302]
          stop <- w263 stop-if-true
          # "Pulse Generator Loop"
          # "usec (16)"
          n55 = Unbundle By Name("Pulse Control") -> ("Loop period (us)"=w291:u16)
          n56 = Unbundle By Name("Pulse Control") -> ("Sample & Hold Period (uSec)"=w295:u32)
          n57 = Unbundle By Name("Pulse Control") -> ("BS Hold ON until"=w290:u32, "BS Hold Delay"=w289:u32, "BS Hold Invert"=w288:bool)
          n58 = Unbundle By Name("Pulse Control") -> ("Probe OFF until"=w287:u32, "Probe Delay"=w286:u32, "Probe Invert"=w285:bool)
          n59 = Unbundle By Name("Pulse Control") -> ("HD ON until"=w284:u32, "HD Delay"=w283:u32, "HD Invert"=w282:bool)
          n60 = Unbundle By Name("Pulse Control") -> ("Measurement ON until"=w281:u32, "Measurement delay"=w280:u32, "Measurement Invert"=w279:bool)
          n61 = xnode "FPGA I/O Node"() -> ("PXI_Trig1"=w259:bool)  [unwired: 1 in, 1 out]
          n62 = xnode "FPGA I/O Node"() -> ("PXI_Trig2"=w258:bool)  [unwired: 1 in, 1 out]
          n63 = Unbundle By Name("Pulse Control") -> ("High Pulse"=w294:i16, "Low Pulse"=w293:i16)
          n64 = call "Loop Timer2"("Count(uSec)"=w291) -> ()  [unwired: 1 out]
          n65 = call "Tick Count"() -> ("Tick Count(uSec)"=w301:u32)
          "Tick Count(uSec)" <- w301
          n66 = Quotient & Remainder(x=w301, y=w295) -> (x-y*floor(x/y)=w296:u32)  [unwired: 1 out]
          n67 = In Range and Coerce(upper limit=w290, x=w296, lower limit=w289) -> (In Range?=w300:bool)  [unwired: 1 out]
          n68 = In Range and Coerce(upper limit=w287, x=w296, lower limit=w286) -> (In Range?=w299:bool)  [unwired: 1 out]
          n69 = In Range and Coerce(upper limit=w284, x=w296, lower limit=w283) -> (In Range?=w297:bool)  [unwired: 1 out]
          n70 = In Range and Coerce(upper limit=w281, x=w296, lower limit=w280) -> (In Range?=w298:bool)  [unwired: 1 out]
          n71 = Exclusive Or(1:w288, 2:w300) -> (0:w275:bool)
          "BS Hold Pulse" <- w275
          n72 = Exclusive Or(1:w285, 2:w299) -> (0:w271:bool)
          "Probe OFF Pulse" <- w271
          n73 = Exclusive Or(1:w282, 2:w297) -> (0:w267:bool)
          "HD Pulse" <- w267
          n74 = Exclusive Or(1:w279, 2:w298) -> (0:w264:bool)
          "Measurment Pulse" <- w264
          n75 = Compound Arithmetic op=OR("stop pulse loop", w259, "Measurement OFF", w258) -> (w261:bool)
          n76 = Select(t=FALSE, s="stop pulse loop", f=w275) -> (s? t:f=w273:bool)
          n77 = Select(t=FALSE, s="stop pulse loop", f=w271) -> (s? t:f=w270:bool)
          n78 = Select(t=FALSE, s="stop pulse loop", f=w267) -> (s? t:f=w268:bool)
          n79 = Select(t=FALSE, s=w261, f=w264) -> (s? t:f=w265:bool)
          n80 = Select(t=w294, s=w273, f=w293) -> (s? t:f=w277:i16)
          n81 = Select(t=w294, s=w270, f=w293) -> (s? t:f=w276:i16)
          n82 = Select(t=w294, s=w268, f=w293) -> (s? t:f=w257:i16)
          n83 = Select(t=w294, s=w265, f=w293) -> (s? t:f=w278:i16)
          n84 = xnode "FPGA I/O Node"("PXI_Trig0"=w273, "Connector0/AO4"=w277, "Connector0/AO5"=w276, "Connector0/AO6"=w257, "Connector0/AO7"=w278) -> ()  [unwired: 5 in, 5 out]
          "Pulse Loop count" <- w302
        }
      }
    }
    "Pulse large loop count" <- w255
  }
  n85 = while {
    i -> [w399]
    stop <- FALSE ("stop") stop-if-true
    # "Scope Loop"
    # "T when state is in \"Scan\" or \"Lock\""
    n86 = local read "Trigger"() -> (w397:T9)
    n87 = Cluster To Array(cluster=w397) -> (array=w401:bool[])
    n88 = Unbundle By Name("Scope") -> ("Channel"=w400:i32)
    n89 = Index Array(array=w401, index=w400) -> (element=w398:bool)
    n90 = case shown="True" w398 {
      tunnel: "Scope" -> [_ w404]
      frame False {
      }
      frame True {
        n91 = flat-sequence {
          tunnel: w404 -> [w405]
          tunnel: [w405] -> w403
          tunnel: w403 -> [w407]
          frame #0 {
            n92 = Unbundle By Name(w405) -> ("Delay"=w406:u32)
            n93 = call "Wait"("Count(Ticks)"=w406) -> ()  [unwired: 1 out]
          }
          frame #1 {
            n94 = for {
              N: 4095 -> [_]
              tunnel: w407 -> [w445]
              shift-right: [w424] -> _
              shift-left: _ -> [w423]
              shift-right: [w419] -> _
              shift-left: _ -> [w418]
              n95 = local read "Cavity Errors"() -> (w444:T11)
              n96 = local read "Outputs"() -> (w443:T8)
              n97 = local read "Cavity Monitors"() -> (w442:T10)
              n98 = local read "Lock Threshold"() -> (w409:T12)
              n99 = xnode ("FIFO Method Node")("Element"=w418, "Timeout"=-1) -> ("Timed Out?"=→"Scope Full?":bool)  [unwired: 1 in, 1 out]
              n100 = Unbundle By Name(w445) -> ("Aquisition Rate (Ticks)"=w446:u32)
              n101 = Unbundle By Name(w445) -> ("Channel Selector.Channel 1"=w420:i32, "Channel Selector.Channel 2"=w421:i32, "Channel Selector.Channel 3"=w411:i32, "Channel Selector.Channel 4"=w422:i32)
              n102 = call "Loop Timer"("Count(uSec)"=w446) -> ()  [unwired: 1 out]
              n103 = Unbundle(w444) -> ("OPO A"=w441:i16, "OPO B"=w440:i16, "MCC"=w439:i16, "Doubler"=w438:i16)
              n104 = Unbundle(w443) -> ("OPO A out"=w437:i16, "OPO B out"=w436:i16, "MCC out"=w435:i16, "Doubler out"=w434:i16)
              n105 = Unbundle(w442) -> ("OPO A Monitor"=w433:i16, "OPO B Monitor"=w432:i16, "MCC Monitor"=w431:i16, "Doubler Monitor"=w430:i16)
              n106 = Unbundle(w409) -> ("Thresh OPO A"=w413:i16, "Thresh OPO B"=w414:i16, "Thresh MCC"=w415:i16, "Thresh Doubler"=w416:i16)
              n107 = Index Array(array=w423, index=w420) -> (element=w426:i16)
              n108 = Index Array(array=w423, index=w421) -> (element=w425:i16)
              n109 = Index Array(array=w423, index=w411) -> (element=w410:i16)
              n110 = Index Array(array=w423, index=w422) -> (element=w427:i16)
              n111 = Join Numbers(hi=w426, lo=w425) -> ((hi.lo)=w429:u32)
              n112 = Join Numbers(hi=w410, lo=w427) -> ((hi.lo)=w428:u32)
              n113 = Build Array(w441, w440, w439, w438, w437, w436, w435, w434, w433, w432, w431, w430, w413, w414, w415, w416) -> (w424:i16[])
              n114 = Join Numbers(hi=w429, lo=w428) -> ((hi.lo)=w419:u64)
            }
          }
        }
      }
    }
    "Scope loop count" <- w399
  }
